vi "SetPacketSize.vi"(3 "错误输入":errorcluster caption="错误输入（无错误）", 4 "IMAQdx Session In":T1, 5 "PacketSize":u32) -> (0 "错误输出":errorcluster, 2 "IMAQdx Session":T1)   [LabVIEW 2012]
uses:
  <vilib>/userDefined/High Color/IMAQdx.ctl
  <resource>/objmgr/imaqdx.rc
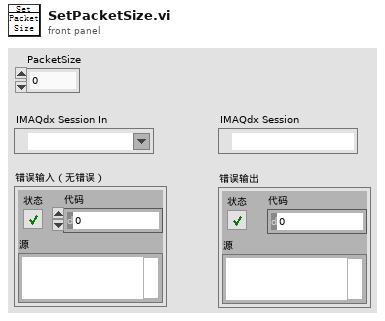
[diagram p1: front panel]
types:
  T1 = typedef "IMAQdx.ctl" = refnum<k21>
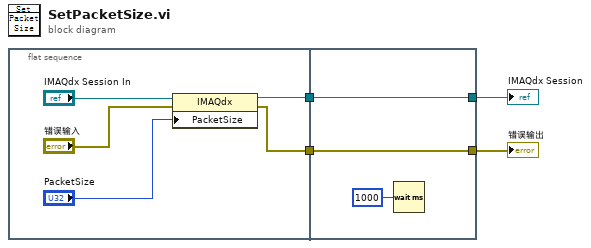
[diagram p0: block diagram]
diagram:
  n1 = flat-sequence {
    tunnel: [w6] -> w4
    tunnel: [w5] -> w3
    tunnel: [w11] -> w1
    tunnel: w4 -> [w11]
    tunnel: [w10] -> w2
    tunnel: w3 -> [w10]
    frame #0 {
      n2 = property class="IMAQdx"(reference="IMAQdx Session In", error in="错误输入", "PacketSize"="PacketSize") -> (reference out=w6:T1, error out=w5:errorcluster)
    }
    frame #1 {
      n3 = Wait (ms)(milliseconds to wait=u32 1000 ("等待时间（毫秒）")) -> ()  [unwired: 1 out]
    }
  }
  "错误输出" <- w2
  "IMAQdx Session" <- w1
